vi "Handlers.vi"(8 "error in (no error)":errorcluster, 9 "Message Loop Shift Register Data":T1, 10 "WAMP Message":T16 {"Message Codes" items=["HELLO"=1, "WELCOME"=2, "ABORT"=3, "GOODBYE"=6, "ERROR"=8, "PUBLISH"=16, "PUBLISHED"=17, "SUBSCRIBE"=32, "SUBSCRIBED"=33, "UNSUBSCRIBE"=34, "UNSUBSCRIBED"=35, "EVENT"=36, "CALL"=48, "RESULT"=59, "REGISTER"=64, "REGISTERED"=65, "UNREGISTER"=66, "UNREGISTERED"=67, "INVOCATION"=68, "YIELD"=70]}, 11 "reference":refnum<class "WAMP Client.lvclass">) -> (0 "error out":errorcluster, 1 "Message Loop Shift Register Data (out)":T1, 3 "reference out":refnum<class "WAMP Client.lvclass">)   [LabVIEW 2020, in "wamplv.lvlib" / "WAMP Client.lvclass"]
uses:
  <vilib>/samangh/wamplv/WAMP Client/WAMP Client.lvclass
  <vilib>/samangh/wamplv/WAMP Client/TypeDef/WAMP Received Message.ctl
  <vilib>/samangh/wamplv/WAMP Message Codes.ctl
  <vilib>/samangh/wamplv/WAMP Client/TypeDef/Message Loop Shift Reg Data.ctl
  <vilib>/samangh/wamplv/WAMP Client/TypeDef/REGISTER Request Data.ctl
  <vilib>/samangh/wamplv/WAMP Client/TypeDef/Success or error.ctl
  <vilib>/samangh/wamplv/WAMP Client/TypeDef/Combined error.ctl
  <vilib>/samangh/wamplv/WAMP Client/TypeDef/WAMP Error Payload.ctl
  <vilib>/samangh/wamplv/WAMP Client/TypeDef/INVOCATION payload.ctl
  <vilib>/samangh/wamplv/WAMP Client/TypeDef/Publish Requests Map.ctl
  <vilib>/samangh/wamplv/WAMP Client/TypeDef/PUBLISH Request Data.ctl
  <vilib>/samangh/wamplv/WAMP Client/TypeDef/PUBLISH Result.ctl
  <vilib>/samangh/wamplv/WAMP Client/TypeDef/Endpoint Data.ctl
  <vilib>/samangh/wamplv/WAMP Client/TypeDef/CALL Request Map.ctl
  <vilib>/samangh/wamplv/WAMP Client/TypeDef/CALL Request Data.ctl
  <vilib>/samangh/wamplv/WAMP Client/TypeDef/RESULT Payload.ctl
  <vilib>/samangh/wamplv/WAMP Client/TypeDef/SUBSCRIBE Requests Map.ctl
  <vilib>/samangh/wamplv/WAMP Client/TypeDef/SUBSCRIBE Request Data.ctl
  <vilib>/samangh/wamplv/WAMP Client/TypeDef/Subscribe Result.ctl
  <vilib>/samangh/wamplv/WAMP Client/TypeDef/Event Payload.ctl
  <vilib>/samangh/wamplv/WAMP Client/TypeDef/Subscriptions Map.ctl
  <vilib>/samangh/wamplv/WAMP Client/TypeDef/Subscription Details.ctl
  <vilib>/samangh/wamplv/WAMP Client/TypeDef/Unsubscribe Requests Map.ctl
  <vilib>/samangh/wamplv/WAMP Client/TypeDef/UNSUBSCRIBE Request Data.ctl
  <vilib>/samangh/wamplv/WAMP Client/TypeDef/UNSUBSCRIBE Result.ctl
  <vilib>/samangh/wamplv/WAMP Client/TypeDef/Unregister requests map.ctl
  <vilib>/samangh/wamplv/WAMP Client/TypeDef/Unregister request.ctl
  <vilib>/samangh/wamplv/WAMP Client/WAMP Client.lvclass/WAMP Client.ctl
  <vilib>/JDP Science/JSONtext/JSONtext.lvlib
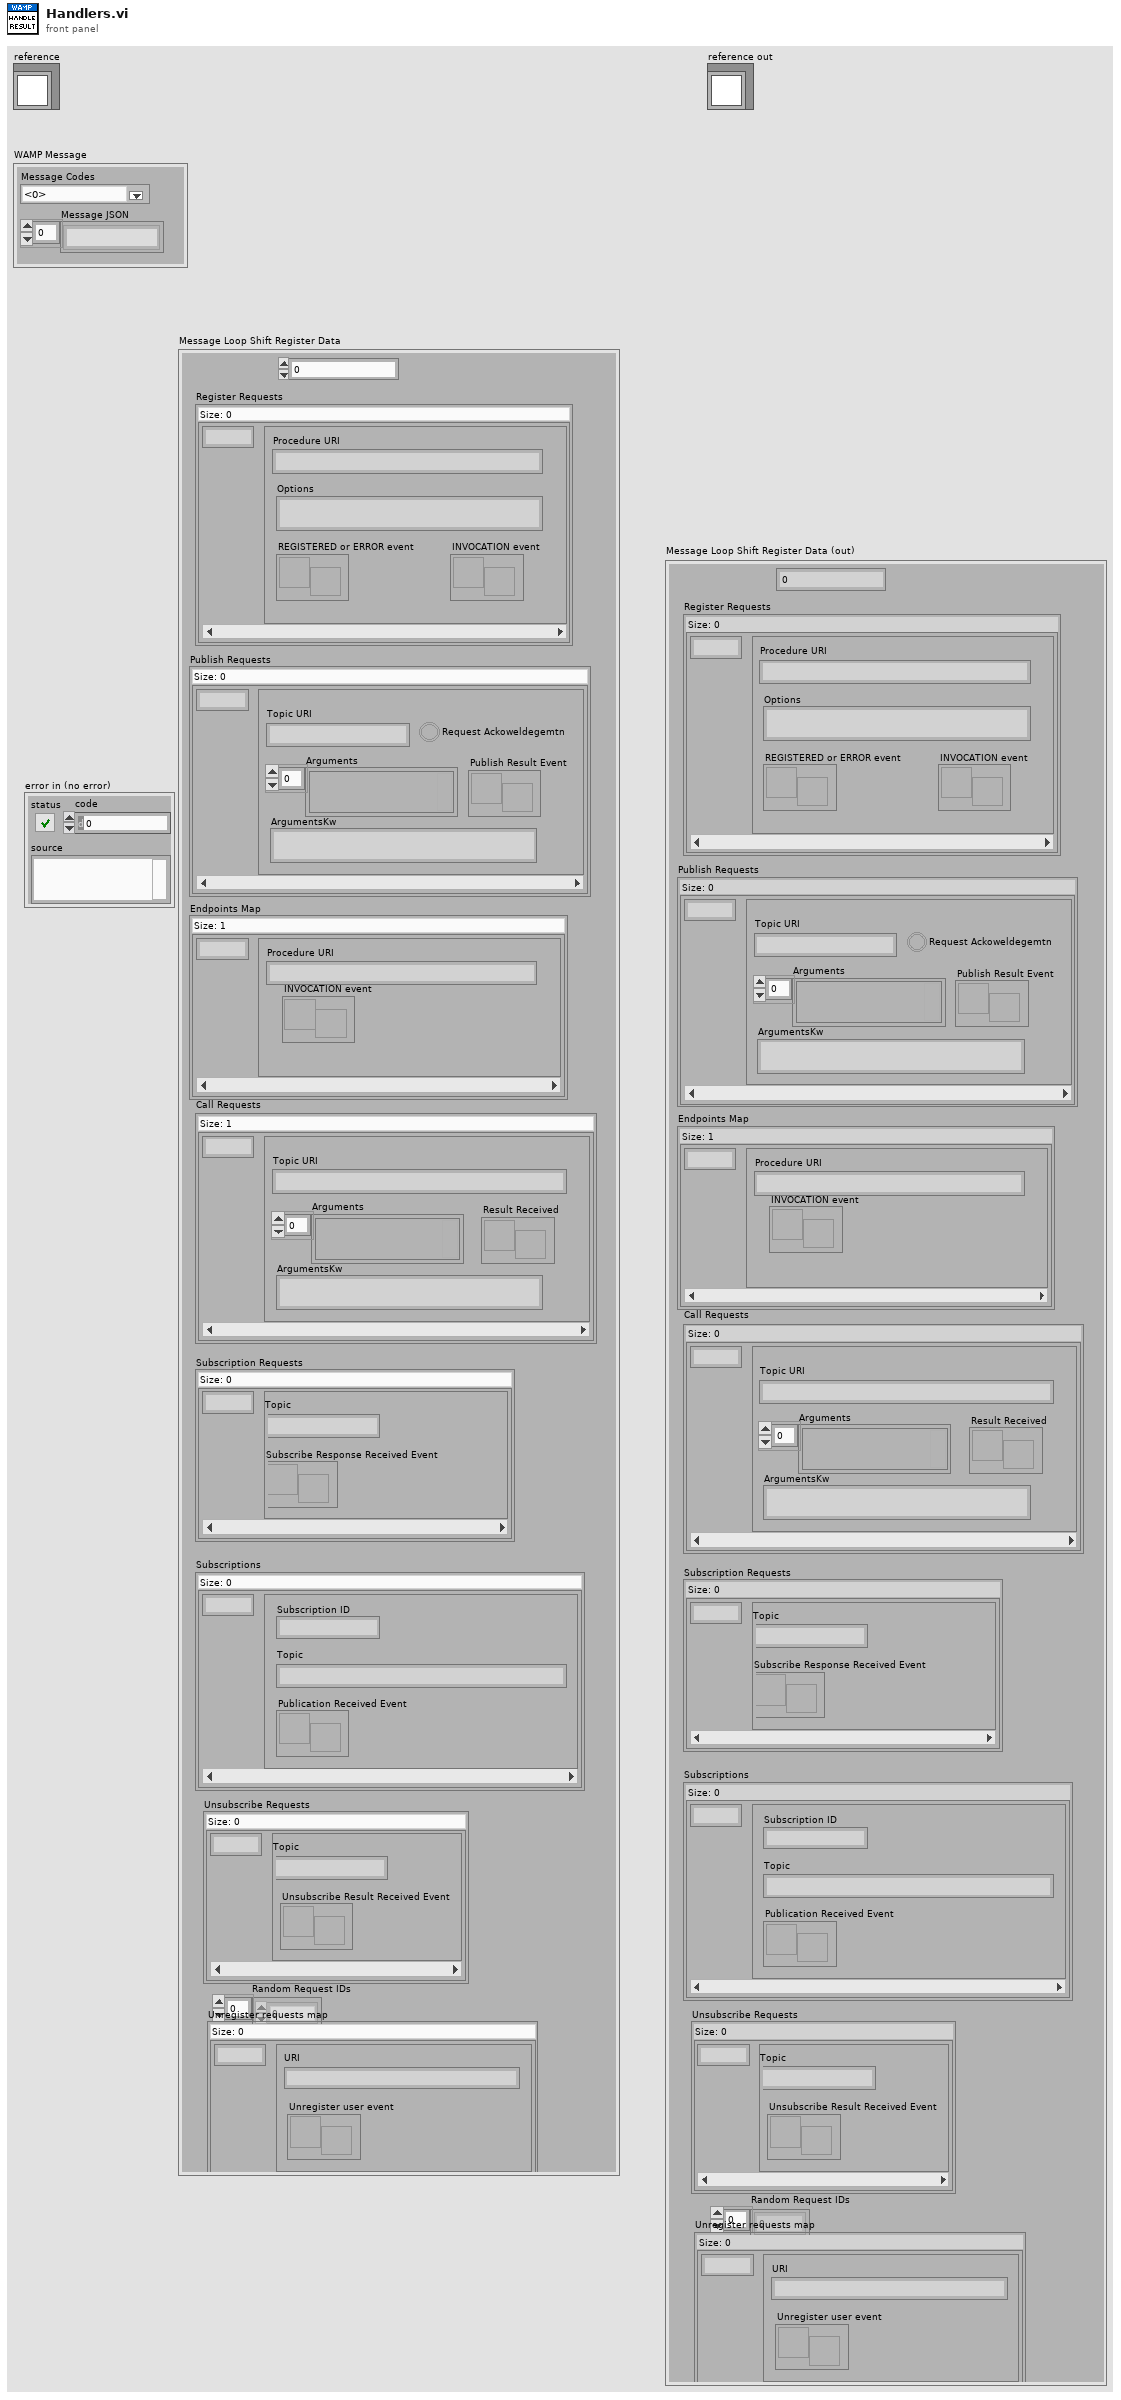
[diagram p1: front panel]
types:
  T1 = typedef "wamplv.lvlib/WAMP Client.lvclass/Message Loop Shift Reg Data.ctl" = cluster{"Last Request ID":u64, "Register Requests":map{u64, T2}, "Publish Requests":T3, "Endpoints Map":map{u64, T5}, "Call Requests":T6, "Subscription Requests":T8, "Subscriptions":T10, "Unsubscribe Requests":T12, "Random Request IDs":u64[], "Unregister requests map":T14}
  T2 = typedef "wamplv.lvlib/WAMP Client.lvclass/REGISTER Request Data.ctl" = cluster{"Procedure URI":string, "Options":string, "REGISTERED or ERROR event":refnum<user-event>, "INVOCATION event":refnum<user-event>}
  T3 = typedef "wamplv.lvlib/WAMP Client.lvclass/Publish Requests Map.ctl" = map{u64, T4}
  T4 = typedef "wamplv.lvlib/WAMP Client.lvclass/PUBLISH Request Data.ctl" = cluster{"Topic URI":string, "Arguments":variant[], "ArgumentsKw":string, "Publish Result Event":refnum<user-event>, "Request Ackoweldegemtn":bool}
  T5 = typedef "wamplv.lvlib/WAMP Client.lvclass/Endpoint Data.ctl" = cluster{"Procedure URI":string, "INVOCATION event":refnum<user-event>}
  T6 = typedef "wamplv.lvlib/WAMP Client.lvclass/CALL Request Map.ctl" = map{u64, T7}
  T7 = typedef "wamplv.lvlib/WAMP Client.lvclass/CALL Request Data.ctl" = cluster{"Topic URI":string, "Arguments":variant[], "ArgumentsKw":string, "Result Received":refnum<user-event>}
  T8 = typedef "wamplv.lvlib/WAMP Client.lvclass/SUBSCRIBE Requests Map.ctl" = map{u64, T9}
  T9 = typedef "wamplv.lvlib/WAMP Client.lvclass/SUBSCRIBE Request Data.ctl" = cluster{"Topic":string, "Subscribe Response Received Event":refnum<user-event>}
  T10 = typedef "wamplv.lvlib/WAMP Client.lvclass/Subscriptions Map.ctl" = map{u64, T11}
  T11 = typedef "wamplv.lvlib/WAMP Client.lvclass/Subscription Details.ctl" = cluster{"Subscription ID":u64, "Topic":string, "Publication Received Event":refnum<user-event>}
  T12 = typedef "wamplv.lvlib/WAMP Client.lvclass/Unsubscribe Requests Map.ctl" = map{u64, T13}
  T13 = typedef "wamplv.lvlib/WAMP Client.lvclass/UNSUBSCRIBE Request Data.ctl" = cluster{"Topic":string, "Unsubscribe Result Received Event":refnum<user-event>}
  T14 = typedef "wamplv.lvlib/WAMP Client.lvclass/Unregister requests map.ctl" = map{u64, T15}
  T15 = typedef "wamplv.lvlib/WAMP Client.lvclass/Unregister request.ctl" = cluster{"URI":string, "Unregister user event":refnum<user-event>}
  T16 = typedef "wamplv.lvlib/WAMP Client.lvclass/WAMP Received Message.ctl" = cluster{"Message JSON":string[], "Message Codes":T17}
  T17 = typedef "wamplv.lvlib/WAMP Client.lvclass/WAMP Message Codes.ctl" = u16
  T18 = typedef "wamplv.lvlib/WAMP Client.lvclass/RESULT Payload.ctl" = cluster{"Arguments Payload":string[], "ArgumentKw Payload":string, "Topic":string, "Success?":bool, "WAMP Error":T19}
  T19 = typedef "wamplv.lvlib/WAMP Client.lvclass/WAMP Error Payload.ctl" = cluster{"Details":string, "ArgumentKw Payload":string, "Wamp error?":bool, "Error URI":string, "Arguments Payload":string[]}
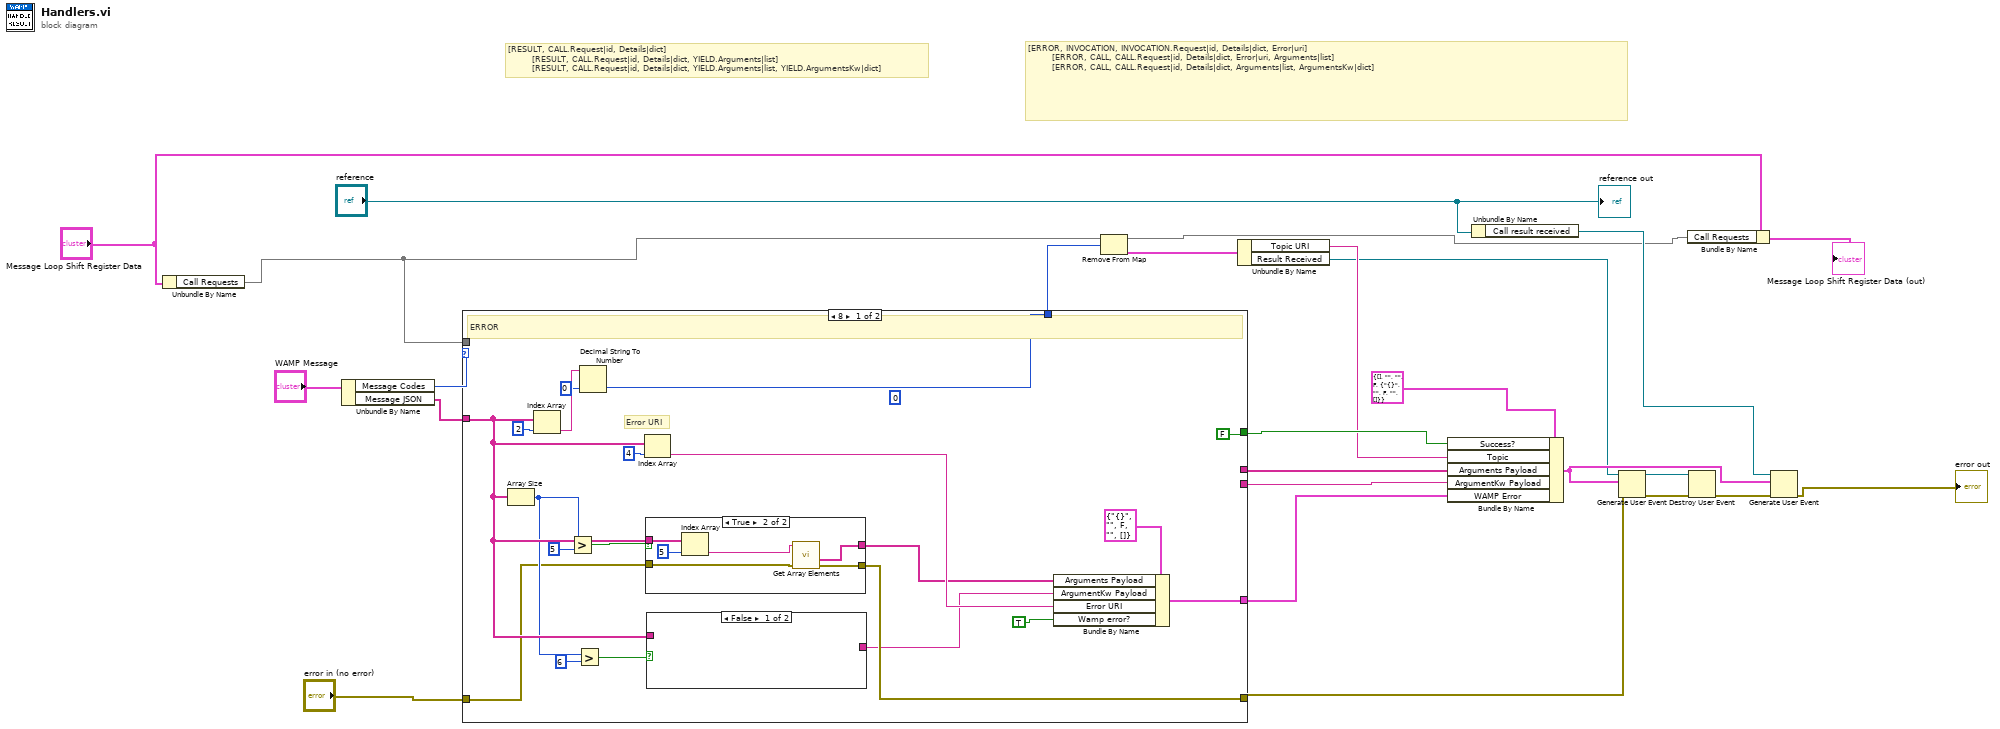
[diagram p0: block diagram]
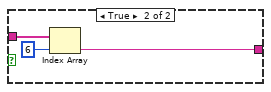
[diagram p2: hidden frame]
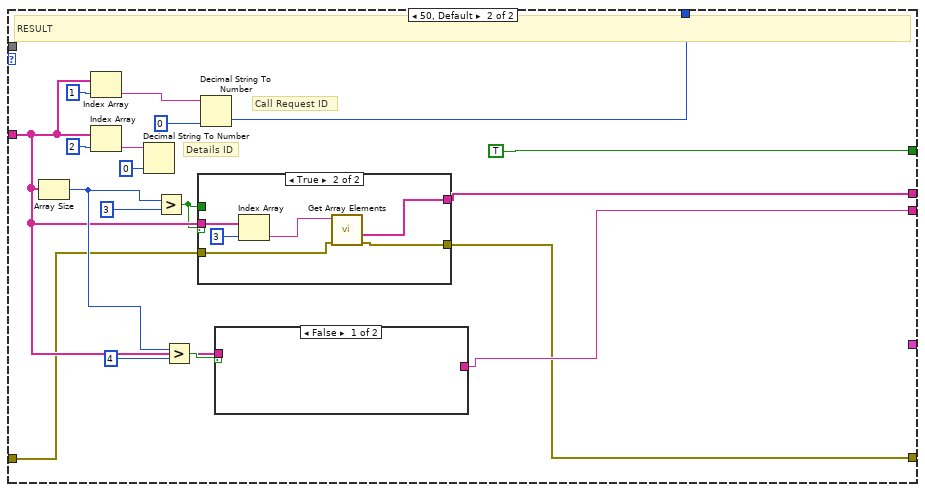
[diagram p4: hidden frame]
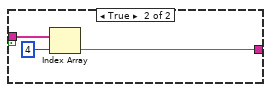
[diagram p5: hidden frame]
diagram:
  # "[ERROR, INVOCATION, INVOCATION.Request|id, Details|dict, Error|uri]\n        [ERROR, CALL, CALL.Request|id, Details|dict, Error|uri, Arguments|list]\n        [ERROR, CALL, CALL.Request|id, Details|dict, Arguments|list, ArgumentsKw|dict]"
  # "[RESULT, CALL.Request|id, Details|dict]\n        [RESULT, CALL.Request|id, Details|dict, YIELD.Arguments|list]\n        [RESULT, CALL.Request|id, Details|dict, YIELD.Arguments|list, YIELD.ArgumentsKw|dict]"
  n1 = Unbundle By Name("Message Loop Shift Register Data") -> ("Call Requests"=w5:T6)
  n2 = Unbundle By Name("WAMP Message") -> ("Message Codes"=w21:T17, "Message JSON"=w20:string[])
  n3 = case shown="8" w21 {
    tunnel: w20 -> [w38 w60]
    tunnel: [w41 w57] -> w19
    tunnel: "error in (no error)" -> [w34 w59]
    tunnel: [w33 w58] -> w23
    tunnel: [FALSE ("Success?") TRUE ("Success?")] -> w24
    tunnel: w5 -> [_ _]
    tunnel: [_ w62] -> w14
    tunnel: [_ w61] -> w13
    tunnel: [w28 _] -> w6
    frame 8 {
      (unwired) 0
      # "Error URI"
      # "ERROR"
      n4 = Array Size(array=w38) -> (size(s)=w35:i32)
      n5 = Index Array(array=w38, index=2) -> (element=w44:string)
      n6 = Greater?(x=w35, y=5) -> (0:w39:bool)
      n7 = Greater?(x=w35, y=6) -> (0:w36:bool)
      n8 = Decimal String To Number(string=w44, default (0L)=u64 0 ("default (0 I32)")) -> (number=w41:u64)  [unwired: 1 in, 1 out]
      n9 = Index Array(array=w38, index=4) -> (element=w30:string)
      n10 = case shown="True" w39 {
        tunnel: w38 -> [_ w54]
        tunnel: w34 -> [w49 w50]
        tunnel: [w49 w51] -> w33
        tunnel: [_ w52] -> w27
        frame False {
        }
        frame True {
          n11 = Index Array(array=w54, index=5) -> (element=w53:string)
          n12 = call <vilib>:"Get Array Elements.vi"("error in (no error)"=w50, "JSON"=w53) -> ("error out"=w51:errorcluster, "<JSON>"=w52:string[])  [unwired: 7 in, 1 out]
        }
      }
      n13 = case shown="False" w36 {
        tunnel: [_ w47] -> w29
        tunnel: w38 -> [_ w46]
        frame False {
        }
        frame True {
          n14 = Index Array(array=w46, index=6) -> (element=w47:string)
        }
      }
      n15 = Bundle By Name(cluster=T19 {"Details"="{}", "ArgumentKw Payload"="", "Wamp error?"=FALSE, "Error URI"="", "Arguments Payload"=[]} ("Cluster"), "Arguments Payload"=w27, "ArgumentKw Payload"=w29, "Error URI"=w30, "Wamp error?"=TRUE ("status")) -> (w28:T19)
    }
    frame 50, Default {
      # "Call Request ID"
      # "Details ID"
      # "RESULT"
      n16 = Array Size(array=w60) -> (size(s)=w63:i32)
      n17 = Index Array(array=w60, index=1) -> (element=w69:string)
      n18 = Index Array(array=w60, index=2) -> (element=w72:string)
      n19 = Decimal String To Number(string=w72, default (0L)=u32 0) -> ()  [unwired: 1 in, 2 out]
      n20 = Greater?(x=w63, y=3) -> (0:w56:bool)
      n21 = Greater?(x=w63, y=4) -> (0:w64:bool)
      n22 = case shown="True" w56 {
        tunnel: w56 -> [_ _]
        tunnel: [_ w82] -> w62
        tunnel: [w77 w81] -> w58
        tunnel: w60 -> [_ w80]
        tunnel: w59 -> [w77 w78]
        frame False {
        }
        frame True {
          n23 = Index Array(array=w80, index=3) -> (element=w79:string)
          n24 = call <vilib>:"Get Array Elements.vi"("error in (no error)"=w78, "JSON"=w79) -> ("error out"=w81:errorcluster, "<JSON>"=w82:string[])  [unwired: 7 in, 1 out]
        }
      }
      n25 = Decimal String To Number(string=w69, default (0L)=u32 0) -> (number=w57:u32)  [unwired: 1 in, 1 out]
      n26 = case shown="False" w64 {
        tunnel: [_ w75] -> w61
        tunnel: w60 -> [_ w74]
        frame False {
        }
        frame True {
          n27 = Index Array(array=w74, index=4) -> (element=w75:string)
        }
      }
    }
  }
  n28 = Remove From Map(10:w19, 11:w5) -> (1:w18:T7, 3:w1:T6)  [unwired: 1 out]
  n29 = Unbundle By Name(w18) -> ("Topic URI"=w12:string, "Result Received"=w4:refnum<user-event>)
  n30 = Bundle By Name(cluster=T18 {"Arguments Payload"=[], "ArgumentKw Payload"="", "Topic"="", "Success?"=FALSE, "WAMP Error"={"Details"="{}", "ArgumentKw Payload"="", "Wamp error?"=FALSE, "Error URI"="", "Arguments Payload"=[]}} ("RESULT Payload"), "Success?"=w24, "Topic"=w12, "Arguments Payload"=w14, "ArgumentKw Payload"=w13, "WAMP Error"=w6) -> (w10:T18)
  n31 = Unbundle By Name("reference") -> ("Call result received"=w9:refnum<user-event>)
  n32 = Generate User Event(user event=w4, event data cluster=w10, error in=w23) -> (user event out=w16:refnum<user-event>, error out=w17:errorcluster)  [unwired: 1 in]
  n33 = Bundle By Name(cluster="Message Loop Shift Register Data", "Call Requests"=w1) -> (→"Message Loop Shift Register Data (out)":T1)
  n34 = Destroy User Event(user event=w16, error in=w17) -> (error out=w8:errorcluster)
  n35 = Generate User Event(user event=w9, event data cluster=w10, error in=w8) -> (error out=→"error out":errorcluster)  [unwired: 1 in, 1 out]
  "reference out" <- "reference"
